vi "create index groupings.vi"(8 "error in":errorcluster, 10 "Create Tags?":bool, 11 "data dictionary":refnum<class "data dictionary.lvclass">) -> (0 "error out":errorcluster, 2 "indices":T1[](array[typedef]))   [LabVIEW 2013, in "CVT runtime.lvclass"]
uses:
  CVT runtime.lvclass
  <vilib>/NI/Current Value Table/Type Defs/Typed Index Set.ctl
  <vilib>/NI/Current Value Table/Type Defs/Data Types.ctl
  <vilib>/NI/Tag Bus/dictionary/data dictionary.lvclass
  <vilib>/NI/Tag Bus/dictionary/data dictionary.lvclass/data dictionary.ctl
  <vilib>/NI/Current Value Table/Type Defs/Single Tag.ctl
  <vilib>/NI/Current Value Table/Type Defs/File Format.ctl
  <vilib>/NI/Current Value Table/Type Defs/Tag Grouping set.ctl
  <vilib>/NI/Current Value Table/Errors/Generate Error.vi
  <vilib>/NI/Current Value Table/FGVs/Tag Memory.vi
  <vilib>/NI/Current Value Table/Current Value Table.lvlib
  <vilib>/NI/Tag Bus/tag/tag descriptor.lvclass
  configuration/CVT configuration.lvclass
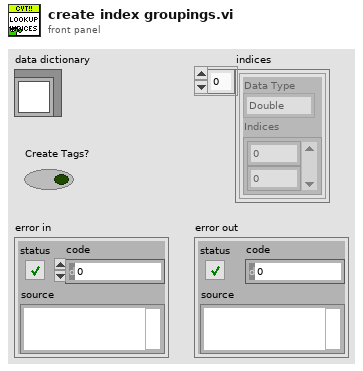
[diagram p1: front panel]
types:
  T1 = typedef "Current Value Table.lvlib/Typed Index Set.ctl" = cluster{"Data Type":T2, "Indices":i32[]}
  T2 = typedef "Current Value Table.lvlib/Data Types.ctl" = enum16{"Double", "Single", "I64", "I32", "I16", "I8", "U64", "U32", "U16", "U8", "String", "Boolean", "Array of U8", "Array of U16", "Array of U32", "Array of U64", "Array of I64", "Array of I32", "Array of I16", "Array of I8", "Array of Double", "Array of Single", "Array of Boolean", "Array of String"}
  T3 = typedef "tag bus.lvlib/data dictionary.lvclass/full data dictionary.ctl" = cluster{"Double":string[], "Single":string[], "I64":string[], "I32":string[], "I16":string[], "I8":string[], "U64":string[], "U32":string[], "U16":string[], "U8":string[], "Boolean":string[], "String":string[], "Array of Double":string[], "Array of Single":string[], "Array of I64":string[], "Array of I32":string[], "Array of I16":string[], "Array of I8":string[], "Array of U64":string[], "Array of U32":string[], "Array of U16":string[], "Array of U8":string[], "Array of Boolean":string[], "Array of String":string[]}
  T4 = typedef "tag bus.lvlib/data table.lvlib/data table.ctl" = cluster{"Double":dbl[], "Single":sgl[], "I64":i64[], "I32":i32[], "I16":i16[], "I8":i8[], "U64":u64[], "U32":u32[], "U16":u16[], "U8":u8[], "Boolean":bool[], "String":string[], "Array of Double":cluster{"DBL Array":dbl[]}[], "Array of Single":cluster{"SGL Array":sgl[]}[], "Array of I64":cluster{"I64 Array":i64[]}[], "Array of I32":cluster{"I32 Array":i32[]}[], "Array of I16":cluster{"I16 Array":i16[]}[], "Array of I8":cluster{"I8 Array":i8[]}[], "Array of U64":cluster{"U64 Array":u64[]}[], "Array of U32":cluster{"U32 Array":u32[]}[], "Array of U16":cluster{"U16 Array":u16[]}[], "Array of U8":cluster{"U8 Array":u8[]}[], "Array of Boolean":cluster{"Boolean Array":bool[]}[], "Array of String":cluster{"String Array":string[]}[]}
  T5 = typedef "Current Value Table.lvlib/Single Tag.ctl" = cluster{"Data Type":T2, "Name":string, "Value":string, "Description":string}
  T6 = typedef "Current Value Table.lvlib/File Format.ctl" = cluster{"Tags":T5[], "Group Listings":T7[]}
  T7 = typedef "Current Value Table.lvlib/Tag Grouping set.ctl" = cluster{"Group":string, "Tag Names":string[]}
  T8 = typedef "tag bus.lvlib/tag descriptor.lvclass/Data Type.ctl" = enum16{"Double", "Single", "I64", "I32", "I16", "I8", "U64", "U32", "U16", "U8", "Boolean", "String", "Array of Double", "Array of Single", "Array of I64", "Array of I32", "Array of I16", "Array of I8", "Array of U64", "Array of U32", "Array of U16", "Array of U8", "Array of Boolean", "Array of String"}
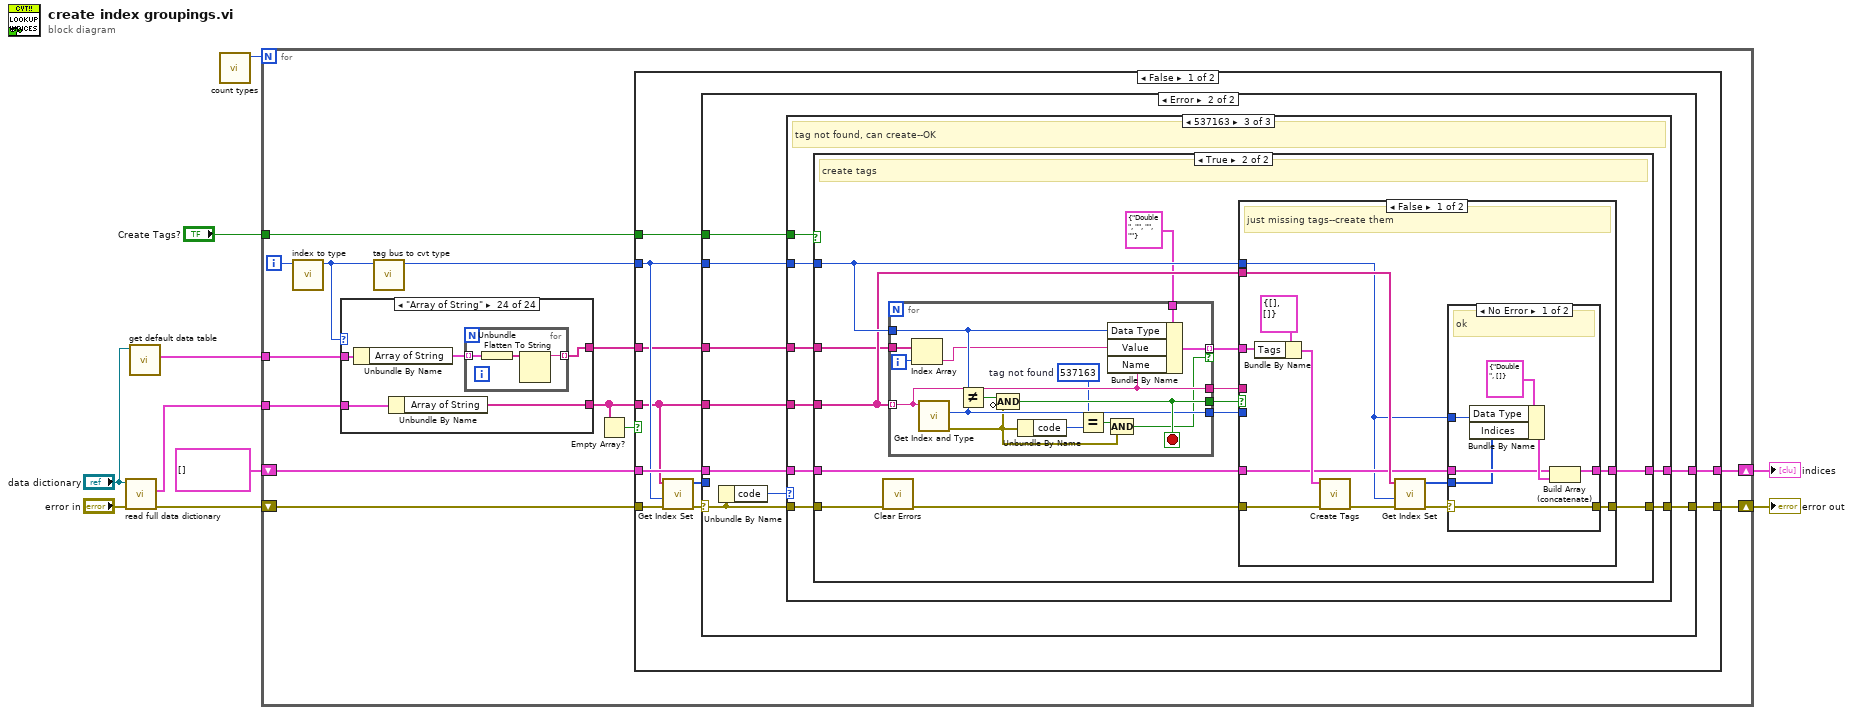
[diagram p0: block diagram]
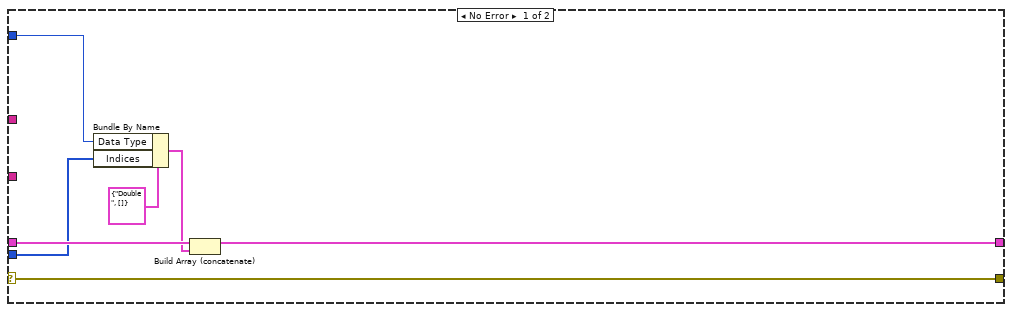
[diagram p2: hidden frame]
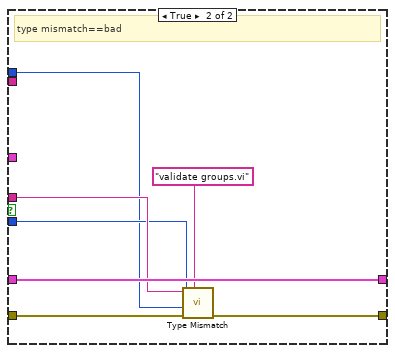
[diagram p7: hidden frame]
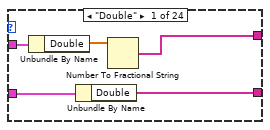
[diagram p9: hidden frame]
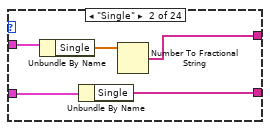
[diagram p10: hidden frame]
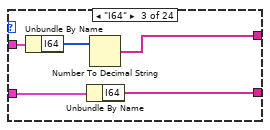
[diagram p11: hidden frame]
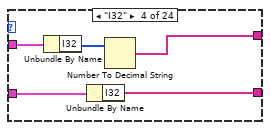
[diagram p12: hidden frame]
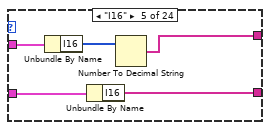
[diagram p13: hidden frame]
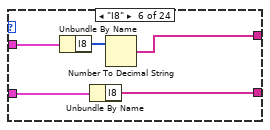
[diagram p14: hidden frame]
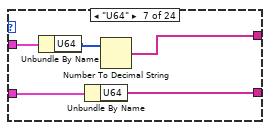
[diagram p15: hidden frame]
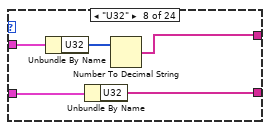
[diagram p16: hidden frame]
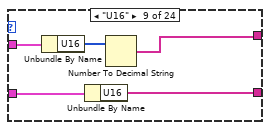
[diagram p17: hidden frame]
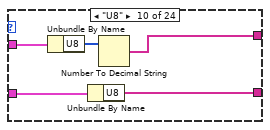
[diagram p18: hidden frame]
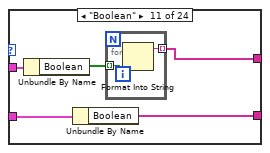
[diagram p19: hidden frame]
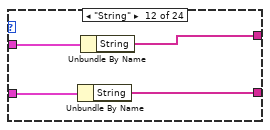
[diagram p20: hidden frame]
diagram:
  n1 = call <vilib>:"read full data dictionary.vi"("error in"="error in", "data dictionary in"="data dictionary") -> ("error out"=w3:errorcluster, "dictionary"=w5:T3)  [unwired: 7 in, 1 out]
  n2 = call <vilib>:"get default data table.vi"("data dictionary in"="data dictionary") -> ("default data table"=w1:T4)  [unwired: 9 in, 1 out]
  n3 = call <vilib>:"count types.vi"() -> ("type count"=w10:i32)  [unwired: 11 in]
  n4 = for {
    N: w10 -> [_]
    shift-right: [w23] -> w8
    shift-left: T1[] [] -> [w22]
    shift-right: [w20] -> w9
    shift-left: w3 -> [w21]
    tunnel: w5 -> [w19]
    tunnel: "Create Tags?" -> [w16]
    tunnel: w1 -> [w14]
    i -> [w15]
    n5 = call <vilib>:"index to type.vi"("I32"=w15) -> ("type"=w12:T8)  [unwired: 10 in]
    n6 = case shown="\"Array of String\"" w12 {
      tunnel: w19 -> [w126 w131 w136 w141 w146 w151 w156 w161 w166 w171 w176 w182 w187 w195 w203 w211 w219 w227 w235 w243 w251 w259 w267 w275]
      tunnel: [w125 w130 w135 w140 w145 w150 w155 w160 w165 w170 w175 w181 w186 w194 w202 w210 w218 w226 w234 w242 w250 w258 w266 w274] -> w18
      tunnel: w14 -> [w124 w129 w134 w139 w144 w149 w154 w159 w164 w169 w174 w180 w184 w193 w201 w209 w215 w225 w233 w241 w249 w257 w265 w273]
      tunnel: [w122 w127 w132 w137 w142 w147 w152 w157 w162 w167 w172 w179 w183 w191 w200 w208 w217 w223 w231 w240 w247 w256 w264 w271] -> w13
      frame "Double" {
        n7 = Unbundle By Name(w124) -> ("Double"=w123:dbl[])
        n8 = Unbundle By Name(w126) -> ("Double"=w125:string[])
        n9 = Number To Fractional String(number=w123) -> (F-format string=w122:string[])  [unwired: 3 in]
      }
      frame "Single" {
        n10 = Unbundle By Name(w129) -> ("Single"=w128:sgl[])
        n11 = Unbundle By Name(w131) -> ("Single"=w130:string[])
        n12 = Number To Fractional String(number=w128) -> (F-format string=w127:string[])  [unwired: 3 in]
      }
      frame "I64" {
        n13 = Unbundle By Name(w134) -> ("I64"=w133:i64[])
        n14 = Unbundle By Name(w136) -> ("I64"=w135:string[])
        n15 = Number To Decimal String(number=w133) -> (decimal integer string=w132:string[])  [unwired: 1 in]
      }
      frame "I32" {
        n16 = Unbundle By Name(w139) -> ("I32"=w138:i32[])
        n17 = Unbundle By Name(w141) -> ("I32"=w140:string[])
        n18 = Number To Decimal String(number=w138) -> (decimal integer string=w137:string[])  [unwired: 1 in]
      }
      frame "I16" {
        n19 = Unbundle By Name(w144) -> ("I16"=w143:i16[])
        n20 = Unbundle By Name(w146) -> ("I16"=w145:string[])
        n21 = Number To Decimal String(number=w143) -> (decimal integer string=w142:string[])  [unwired: 1 in]
      }
      frame "I8" {
        n22 = Unbundle By Name(w149) -> ("I8"=w148:i8[])
        n23 = Unbundle By Name(w151) -> ("I8"=w150:string[])
        n24 = Number To Decimal String(number=w148) -> (decimal integer string=w147:string[])  [unwired: 1 in]
      }
      frame "U64" {
        n25 = Unbundle By Name(w154) -> ("U64"=w153:u64[])
        n26 = Unbundle By Name(w156) -> ("U64"=w155:string[])
        n27 = Number To Decimal String(number=w153) -> (decimal integer string=w152:string[])  [unwired: 1 in]
      }
      frame "U32" {
        n28 = Unbundle By Name(w159) -> ("U32"=w158:u32[])
        n29 = Unbundle By Name(w161) -> ("U32"=w160:string[])
        n30 = Number To Decimal String(number=w158) -> (decimal integer string=w157:string[])  [unwired: 1 in]
      }
      frame "U16" {
        n31 = Unbundle By Name(w164) -> ("U16"=w163:u16[])
        n32 = Unbundle By Name(w166) -> ("U16"=w165:string[])
        n33 = Number To Decimal String(number=w163) -> (decimal integer string=w162:string[])  [unwired: 1 in]
      }
      frame "U8" {
        n34 = Unbundle By Name(w169) -> ("U8"=w168:u8[])
        n35 = Unbundle By Name(w171) -> ("U8"=w170:string[])
        n36 = Number To Decimal String(number=w168) -> (decimal integer string=w167:string[])  [unwired: 1 in]
      }
      frame "Boolean" {
        n37 = Unbundle By Name(w174) -> ("Boolean"=w173:bool[])
        n38 = Unbundle By Name(w176) -> ("Boolean"=w175:string[])
        n39 = for {
          tunnel: w173 -> [w178] mode=indexing
          tunnel: [w177] -> w172 mode=indexing
          n40 = Format Into String(w178) -> (resulting string=w177:string)  [unwired: 3 in, 1 out]
        }
      }
      frame "String" {
        n41 = Unbundle By Name(w182) -> ("String"=w181:string[])
        n42 = Unbundle By Name(w180) -> ("String"=w179:string[])
      }
      frame "Array of Double" {
        n43 = Unbundle By Name(w184) -> ("Array of Double"=w185:cluster{"DBL Array":dbl[]}[])
        n44 = Unbundle By Name(w187) -> ("Array of Double"=w186:string[])
        n45 = for {
          tunnel: w185 -> [w190] mode=indexing
          tunnel: [w188] -> w183 mode=indexing
          n46 = Unbundle(w190) -> ("DBL Array"=w189:dbl[])
          n47 = Flatten To String(anything=w189) -> (data string=w188:string)  [unwired: 3 in, 2 out]
        }
      }
      frame "Array of Single" {
        n48 = Unbundle By Name(w193) -> ("Array of Single"=w192:cluster{"SGL Array":sgl[]}[])
        n49 = Unbundle By Name(w195) -> ("Array of Single"=w194:string[])
        n50 = for {
          tunnel: w192 -> [w198] mode=indexing
          tunnel: [w196] -> w191 mode=indexing
          n51 = Unbundle(w198) -> ("SGL Array"=w197:sgl[])
          n52 = Flatten To String(anything=w197) -> (data string=w196:string)  [unwired: 3 in, 2 out]
        }
      }
      frame "Array of I64" {
        n53 = Unbundle By Name(w201) -> ("Array of I64"=w199:cluster{"I64 Array":i64[]}[])
        n54 = Unbundle By Name(w203) -> ("Array of I64"=w202:string[])
        n55 = for {
          tunnel: w199 -> [w206] mode=indexing
          tunnel: [w204] -> w200 mode=indexing
          n56 = Unbundle(w206) -> ("I64 Array"=w205:i64[])
          n57 = Flatten To String(anything=w205) -> (data string=w204:string)  [unwired: 3 in, 2 out]
        }
      }
      frame "Array of I32" {
        n58 = Unbundle By Name(w209) -> ("Array of I32"=w207:cluster{"I32 Array":i32[]}[])
        n59 = Unbundle By Name(w211) -> ("Array of I32"=w210:string[])
        n60 = for {
          tunnel: w207 -> [w214] mode=indexing
          tunnel: [w212] -> w208 mode=indexing
          n61 = Unbundle(w214) -> ("I32 Array"=w213:i32[])
          n62 = Flatten To String(anything=w213) -> (data string=w212:string)  [unwired: 3 in, 2 out]
        }
      }
      frame "Array of I16" {
        n63 = Unbundle By Name(w215) -> ("Array of I16"=w216:cluster{"I16 Array":i16[]}[])
        n64 = Unbundle By Name(w219) -> ("Array of I16"=w218:string[])
        n65 = for {
          tunnel: w216 -> [w222] mode=indexing
          tunnel: [w220] -> w217 mode=indexing
          n66 = Unbundle(w222) -> ("I16 Array"=w221:i16[])
          n67 = Flatten To String(anything=w221) -> (data string=w220:string)  [unwired: 3 in, 2 out]
        }
      }
      frame "Array of I8" {
        n68 = Unbundle By Name(w225) -> ("Array of I8"=w224:cluster{"I8 Array":i8[]}[])
        n69 = Unbundle By Name(w227) -> ("Array of I8"=w226:string[])
        n70 = for {
          tunnel: w224 -> [w230] mode=indexing
          tunnel: [w228] -> w223 mode=indexing
          n71 = Unbundle(w230) -> ("I8 Array"=w229:i8[])
          n72 = Flatten To String(anything=w229) -> (data string=w228:string)  [unwired: 3 in, 2 out]
        }
      }
      frame "Array of U64" {
        n73 = Unbundle By Name(w233) -> ("Array of U64"=w232:cluster{"U64 Array":u64[]}[])
        n74 = Unbundle By Name(w235) -> ("Array of U64"=w234:string[])
        n75 = for {
          tunnel: w232 -> [w238] mode=indexing
          tunnel: [w236] -> w231 mode=indexing
          n76 = Unbundle(w238) -> ("U64 Array"=w237:u64[])
          n77 = Flatten To String(anything=w237) -> (data string=w236:string)  [unwired: 3 in, 2 out]
        }
      }
      frame "Array of U32" {
        n78 = Unbundle By Name(w241) -> ("Array of U32"=w239:cluster{"U32 Array":u32[]}[])
        n79 = Unbundle By Name(w243) -> ("Array of U32"=w242:string[])
        n80 = for {
          tunnel: w239 -> [w246] mode=indexing
          tunnel: [w244] -> w240 mode=indexing
          n81 = Unbundle(w246) -> ("U32 Array"=w245:u32[])
          n82 = Flatten To String(anything=w245) -> (data string=w244:string)  [unwired: 3 in, 2 out]
        }
      }
      frame "Array of U16" {
        n83 = Unbundle By Name(w249) -> ("Array of U16"=w248:cluster{"U16 Array":u16[]}[])
        n84 = Unbundle By Name(w251) -> ("Array of U16"=w250:string[])
        n85 = for {
          tunnel: w248 -> [w254] mode=indexing
          tunnel: [w252] -> w247 mode=indexing
          n86 = Unbundle(w254) -> ("U16 Array"=w253:u16[])
          n87 = Flatten To String(anything=w253) -> (data string=w252:string)  [unwired: 3 in, 2 out]
        }
      }
      frame "Array of U8" {
        n88 = Unbundle By Name(w257) -> ("Array of U8"=w255:cluster{"U8 Array":u8[]}[])
        n89 = Unbundle By Name(w259) -> ("Array of U8"=w258:string[])
        n90 = for {
          tunnel: w255 -> [w262] mode=indexing
          tunnel: [w260] -> w256 mode=indexing
          n91 = Unbundle(w262) -> ("U8 Array"=w261:u8[])
          n92 = Flatten To String(anything=w261) -> (data string=w260:string)  [unwired: 3 in, 2 out]
        }
      }
      frame "Array of Boolean" {
        n93 = Unbundle By Name(w265) -> ("Array of Boolean"=w263:cluster{"Boolean Array":bool[]}[])
        n94 = Unbundle By Name(w267) -> ("Array of Boolean"=w266:string[])
        n95 = for {
          tunnel: w263 -> [w270] mode=indexing
          tunnel: [w268] -> w264 mode=indexing
          n96 = Unbundle(w270) -> ("Boolean Array"=w269:bool[])
          n97 = Flatten To String(anything=w269) -> (data string=w268:string)  [unwired: 3 in, 2 out]
        }
      }
      frame "Array of String" {
        n98 = Unbundle By Name(w273) -> ("Array of String"=w272:cluster{"String Array":string[]}[])
        n99 = Unbundle By Name(w275) -> ("Array of String"=w274:string[])
        n100 = for {
          tunnel: w272 -> [w278] mode=indexing
          tunnel: [w276] -> w271 mode=indexing
          n101 = Unbundle(w278) -> ("String Array"=w277:string[])
          n102 = Flatten To String(anything=w277) -> (data string=w276:string)  [unwired: 3 in, 2 out]
        }
      }
    }
    n103 = call "tag bus to cvt type.vi"("Data Type"=w12) -> ("cvt type"=w11:T2)  [unwired: 10 in]
    n104 = Empty Array?(array=w18) -> (empty?=w17:bool)
    n105 = case shown="False" w17 {
      tunnel: [w33 w121] -> w23
      tunnel: w22 -> [w32 w121]
      tunnel: w21 -> [w31 w120]
      tunnel: [w30 w120] -> w20
      tunnel: w11 -> [w27 _]
      tunnel: w18 -> [w26 _]
      tunnel: w16 -> [w25 _]
      tunnel: w13 -> [w24 _]
      frame False {
        n106 = call <vilib>:"Get Index Set.vi"("error in (no error)"=w31, "Expected Type"=w27, "Tag Names"=w26) -> ("error out"=w29:errorcluster, "Tag References"=w28:i32[])  [unwired: 7 in]
        n107 = case shown="Error" w29 {
          selector: w29 -> [w40 w46]
          tunnel: [w40 w47] -> w30
          tunnel: w32 -> [w38 w49]
          tunnel: [w37 w48] -> w33
          tunnel: w27 -> [w35 w44]
          tunnel: w28 -> [w34 _]
          tunnel: w26 -> [_ w45]
          tunnel: w25 -> [_ w42]
          tunnel: w24 -> [_ w41]
          frame No Error {
            n108 = Bundle By Name(cluster=T1 {"Data Type"=enum."Double", "Indices"=[]} ("Index Type Set"), "Data Type"=w35, "Indices"=w34) -> (w36:T1)
            n109 = Build Array (concatenate)(w38, w36) -> (w37:T1[])
          }
          frame Error {
            n110 = Unbundle By Name(w46) -> ("code"=w43:i32)
            n111 = case shown="537163" w43 {
              tunnel: w49 -> [w50 w53 w58]
              tunnel: [w50 w53 w59] -> w48
              tunnel: [w51 w52 w60] -> w47
              tunnel: w46 -> [w51 w52 w61]
              tunnel: w45 -> [_ _ w56]
              tunnel: w44 -> [_ _ w57]
              tunnel: w42 -> [_ _ w55]
              tunnel: w41 -> [_ _ w54]
              frame Default {
                # "unk"
              }
              frame 537165 {
                # "tag found but type mismatch"
              }
              frame 537163 {
                # "tag not found, can create--OK"
                n112 = case shown="True" w55 {
                  tunnel: w61 -> [w63 w76]
                  tunnel: [w63 w74] -> w60
                  tunnel: [w62 w73] -> w59
                  tunnel: w58 -> [w62 w72]
                  tunnel: w57 -> [_ w68]
                  tunnel: w56 -> [_ w66]
                  tunnel: w54 -> [_ w64]
                  frame False {
                    # "do not create tags"
                  }
                  frame True {
                    # "create tags"
                    n113 = call <vilib>:"Clear Errors.vi"("error in (no error)"=w76) -> ("error out"=w75:errorcluster)  [unwired: 6 in]
                    n114 = for {
                      tunnel: w66 -> [w114] mode=indexing
                      tunnel: w68 -> [w115]
                      tunnel: [w118] -> w71
                      tunnel: [w114] -> w70
                      tunnel: [w117] -> w69
                      tunnel: [w116] -> w67 mode=indexing if=w105
                      tunnel: T5 {"Data Type"=enum."Double", "Name"="", "Value"="", "Description"=""} ("Tag") -> [w111]
                      tunnel: w64 -> [w110]
                      i -> [w108]
                      stop <- w118 stop-if-true
                      w112 = 537163  # tag not found
                      n115 = Index Array(array=w110, index=w108) -> (element=w109:string)
                      n116 = call <vilib>:"Get Index and Type.vi"("Tag"=w114) -> ("error out"=w107:errorcluster, "Type"=w117:T2)  [unwired: 8 in, 1 out]
                      n117 = Not Equal?(x=w115, y=w117) -> (x != y?=w119:bool)
                      n118 = Compound Arithmetic op=AND(w119, invert w107) -> (w118:bool)
                      n119 = Unbundle By Name(w107) -> ("code"=w113:i32)
                      n120 = Equal?(x=w112, y=w113) -> (x = y?=w106:bool)
                      n121 = Bundle By Name(cluster=w111, "Data Type"=w115, "Value"=w109, "Name"=w114) -> (w116:T5)
                      n122 = Compound Arithmetic op=AND(w106, w107) -> (w105:bool)
                    }
                    n123 = case shown="False" w71 {
                      tunnel: w75 -> [w88 w104]
                      tunnel: [w84 w103] -> w74
                      tunnel: [w79 w102] -> w73
                      tunnel: w72 -> [w80 w102]
                      tunnel: w70 -> [_ w101]
                      tunnel: w69 -> [_ w100]
                      tunnel: w68 -> [w78 w99]
                      tunnel: w67 -> [w85 _]
                      tunnel: w66 -> [w82 _]
                      frame False {
                        # "just missing tags--create them"
                        n124 = Bundle By Name(cluster=T6 {"Tags"=[], "Group Listings"=[]} ("CVT Tags to Create"), "Tags"=w85) -> (w86:T6)
                        n125 = call <vilib>:"Create Tags.vi"("error in (no error)"=w88, "CVT Tags to Create"=w86) -> ("error out"=w83:errorcluster)  [unwired: 9 in]
                        n126 = call <vilib>:"Get Index Set.vi"("error in (no error)"=w83, "Expected Type"=w78, "Tag Names"=w82) -> ("error out"=w81:errorcluster, "Tag References"=w77:i32[])  [unwired: 7 in]
                        n127 = case shown="No Error" w81 {
                          selector: w81 -> [w95 w97]
                          tunnel: [w95 w97] -> w84
                          tunnel: w80 -> [w92 w96]
                          tunnel: [w91 w96] -> w79
                          tunnel: w78 -> [w90 _]
                          tunnel: w77 -> [w89 _]
                          frame No Error {
                            # "ok"
                            n128 = Bundle By Name(cluster=T1 {"Data Type"=enum."Double", "Indices"=[]} ("Index Type Set"), "Data Type"=w90, "Indices"=w89) -> (w93:T1)
                            n129 = Build Array (concatenate)(w92, w93) -> (w91:T1[])
                          }
                          frame Error {
                            # "unk"
                          }
                        }
                      }
                      frame True {
                        # "type mismatch==bad"
                        n130 = call <vilib>:"Type Mismatch.vi"("caller name"="validate groups.vi", "error in (no error)"=w104, "Data Type Requested"=w99, "True Type"=w100, "Tag"=w101) -> ("error out"=w103:errorcluster)  [unwired: 6 in]
                      }
                    }
                  }
                }
              }
            }
          }
        }
      }
      frame True {
      }
    }
  }
  "error out" <- w9
  "indices" <- w8
